vi "WaveformCheck.vi"(8 "error in (no error)":errorcluster, 11 "Class In":refnum<class "ScopePluginsBase.lvclass">) -> (0 "error out":errorcluster, 1 "Run?":bool, 2 "Continuous":bool, 3 "Class Out":refnum<class "ScopePluginsBase.lvclass">)   [LabVIEW 2018, in "ScopePlugins.lvlib"]
uses:
  ScopePlugins.lvlib
  ScopePluginBaseClass/ScopePluginsBase.lvclass
  ScopePluginBaseClass/ScopePluginsBase.lvclass/ScopePluginsBase.ctl
  ScopePluginBaseClass/Accessors/Read Acquisition.vi
  ScopePluginBaseClass/Accessors/Read Channels.vi
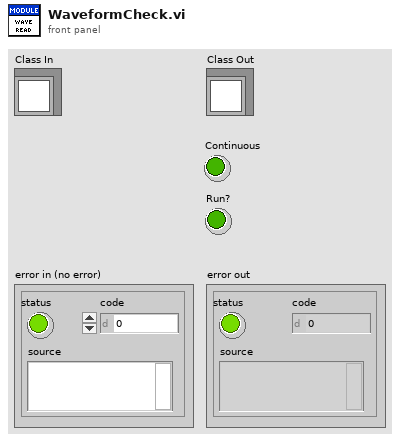
[diagram p1: front panel]
types:
  T1 = typedef "ScopePlugins.lvlib/Acquisition.ctl" = cluster{"StartTime":dbl, "Type":enum16{"Normal", "PeakDetect", "HighRes", "Envelope", "Average"}, "NumPointsMin":i32, "RecordLength":i32, "SampleRate":dbl, "TimePerRecord":dbl, "SamplingMode ":enum16{"Real Time", "Equivalent Time", "Segment", "Real Time Peak Detect", "Real Time High Resolution", "Peak Detect Segment", "High Resolution Segment"}, "Interpolation":enum16{"No Interpolation", "sin(x)/x", "linear", "1 Point sin(x)/x", "2 Point sin(x)/x", "4 Point sin(x)/x", "8 Point sin(x)/x", "16 Point sin(x)/x"}, "NumAverages":i32, "Resolution":enum16{"Auto", "Bits 9", "Bits 10", "Bits 11", "Bits 12"}, "EnableAveraging":bool, "Continuous":bool}
  T2 = typedef "ScopePlugins.lvlib/Channels.ctl" = cluster{"Count":i32, "ChannelArray":T3[]}
  T3 = typedef "ScopePlugins.lvlib/Channel.ctl" = cluster{"Enabled":bool, "Name":string, "InputImpedance":dbl, "InputFreqMax":dbl, "ProbeAttn":dbl, "Coupling":enum16{"AC", "DC", "GND"}, "Offset":dbl, "Range":dbl, "Handle":string, "Connected":bool, "Options String ":string}
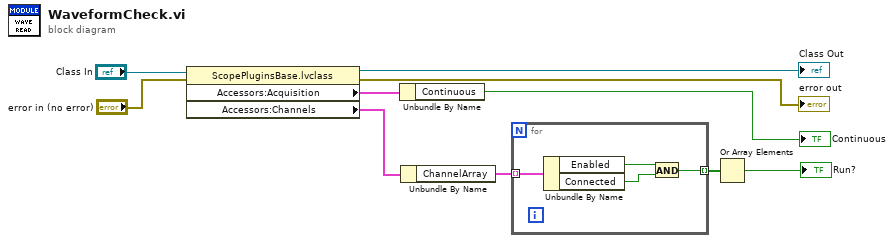
[diagram p0: block diagram]
diagram:
  n1 = property class="ScopePluginsBase.lvclass"(reference="Class In", error in="error in (no error)") -> (reference out=→"Class Out":refnum<class "ScopePluginsBase.lvclass">, error out=→"error out":errorcluster, "Accessors:Acquisition"=w7:T1, "Accessors:Channels"=w8:T2)
  n2 = Unbundle By Name(w7) -> ("Continuous"=→"Continuous":bool)
  n3 = Unbundle By Name(w8) -> ("ChannelArray"=w10:T3[])
  n4 = for {
    tunnel: w10 -> [w14] mode=indexing
    tunnel: [w11] -> w9 mode=indexing
    n5 = Unbundle By Name(w14) -> ("Enabled"=w13:bool, "Connected"=w12:bool)
    n6 = And(x=w13, y=w12) -> (x .and. y?=w11:bool)
  }
  n7 = Or Array Elements(Boolean array=w9) -> (logical OR=→"Run?":bool)
